vi "(RAG) Load Markdown into KB.vi"(0 "Python Session Refnum in":refnum<k35>, 1 "Chroma Database Folder":path, 2 "Knowledge Base Name":string, 3 "Clear DB?":bool=TRUE, 5 "Markdown Folder to Build KB":path, 7 "Chunk Settings":T1={"Chunk Size"=1000, "Chunk Overlap"=100}, 9 "Separators":string="\"\\n## \", \"\\n### \", \"\\n#### \", \"\\n\", \" \", \"\"", 11 "error in":errorcluster, 12 "Embedding Model Base URL":string, 13 "Embedding Model":string) -> (4 "Python Session Refnum out":refnum<k35>, 15 "error out":errorcluster)   [LabVIEW 2023, in "LabVIEW RAG.lvlib"]
uses:
  LabVIEW RAG.lvlib
  Typedefs/RAG Chunk Settings.ctl
  AI RAG Globals.vi
  labview-ai-share/LabVIEW AI Base.lvlib
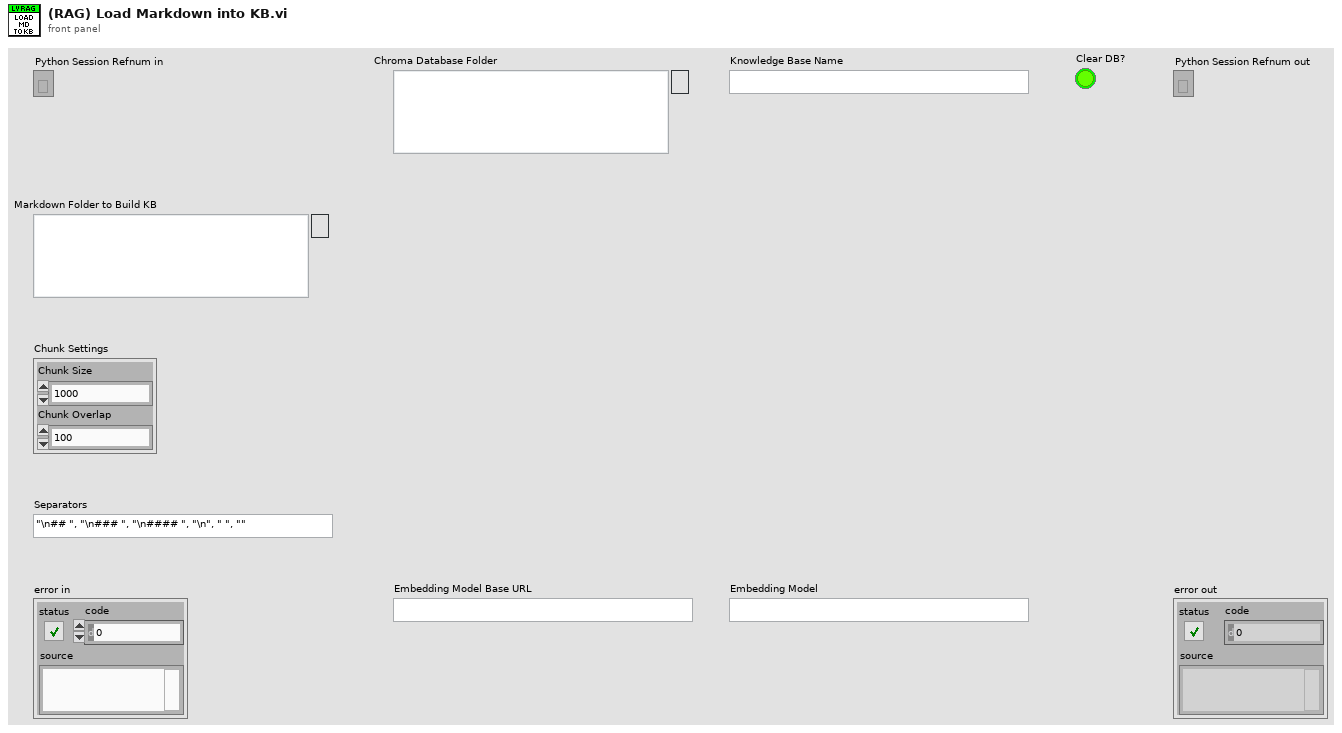
[diagram p1: front panel]
types:
  T1 = typedef "LabVIEW RAG.lvlib/RAG Chunk Settings.ctl" = cluster{"Chunk Size":u32, "Chunk Overlap":u32}
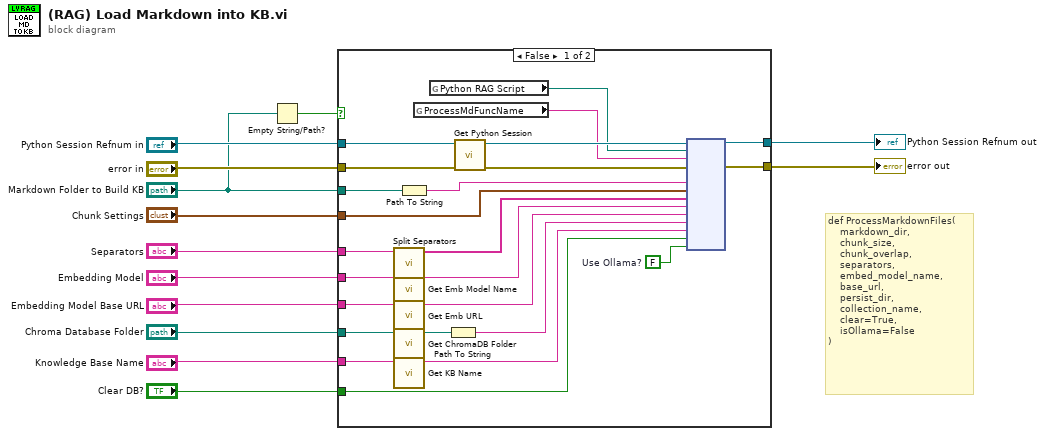
[diagram p0: block diagram]
diagram:
  # "def ProcessMarkdownFiles(\n    markdown_dir, \n    chunk_size, \n    chunk_overlap, \n    separators, \n    embed_model_name, \n    base_url, \n    persist_dir, \n    collection_name, \n    clear=True, \n    isOllama=False\n)"
  n1 = Empty String/Path?(string/path="Markdown Folder to Build KB") -> (empty?=w2:bool)
  n2 = case shown="False" w2 {
    tunnel: "Knowledge Base Name" -> [w36 _]
    tunnel: "Embedding Model Base URL" -> [w35 _]
    tunnel: "Embedding Model" -> [w34 _]
    tunnel: "Chroma Database Folder" -> [w33 _]
    tunnel: [w31 w37] -> w9
    tunnel: "Markdown Folder to Build KB" -> [w30 _]
    tunnel: [w29 w38] -> w8
    tunnel: "error in" -> [w28 w38]
    tunnel: "Python Session Refnum in" -> [w27 w37]
    tunnel: "Chunk Settings" -> [w22 _]
    tunnel: "Clear DB?" -> [w17 _]
    tunnel: "Separators" -> [w14 _]
    frame False {
      w16 = FALSE  # Use Ollama?
      n3 = call "Split Separators.vi"("Separators"=w14) -> ("Separator List"=w15:string[])  [unwired: 10 in]
      n4 = call "Get Emb Model Name.vi"("Embedding Model Name in"=w34) -> ("Embedding Model Name out"=w21:string)  [unwired: 10 in]
      n5 = call "Get Emb URL.vi"("Embedding Model URL in"=w35) -> ("Embedding Model URL out"=w20:string)  [unwired: 10 in]
      n6 = call "Get ChromaDB Folder.vi"("ChromaDB Folder in"=w33) -> ("ChromaDB Folder out"=w25:path)  [unwired: 10 in]
      n7 = call "Get KB Name.vi"("KB Name"=w36) -> ("KB Name"=w18:string)  [unwired: 10 in]
      n8 = Path To String(path=w30) -> (string=w32:string)
      n9 = global read "AI RAG Globals.vi" "ProcessMdFuncName"() -> (w24:string)
      n10 = global read "AI RAG Globals.vi" "Python RAG Script"() -> (w23:path)
      n11 = Path To String(path=w25) -> (string=w19:string)
      n12 = call "Get Python Session.vi"("Python Session in"=w27) -> ("Python Session out"=w26:refnum<k35>)  [unwired: 10 in]
      n13 = node(w26, w23, w24, w28, w32, w22, w15, w21, w20, w19, w18, w17, w16) -> (w31:refnum<k35>, w29:errorcluster)  [unwired: 11 in, 2 out]
    }
    frame True {
    }
  }
  "Python Session Refnum out" <- w9
  "error out" <- w8
